vi "QPSK-PrError.vi"() -> ()   [LabVIEW 2019]
panel:
  out "Histogram":dynamicdata(graph)
  out "Sigma v.s. Eb/N0":cluster{"Y":dbl[], "Y":dbl[]}[](graph)=[{"Y"=[-4.0, -3.0, -2.0, -1.0, 0.0, 1.0, 2.0, 3.0, 4.0, 5.0, 6.0, 7.0, 8.0, 9.0, 10.0], "Y"=[0.22360679774997896, 0.22360679774997896, 0.22360679774997896, 0.22360679774997896, 0.22360679774997896, 0.22360679774997896, 0.22360679774997896, 0.22360679774997896, 0.22360679774997896, 0.22360679774997896, 0.22360679774997896, 0.22360679774997896, 0.22360679774997896, 0.22360679774997896, 0.22360679774997896]}, {"Y"=[-4.0, -3.0, -2.0, -1.0, 0.0, 1.0, 2.0, 3.0, 4.0, 5.0, 6.0, 7.0, 8.0, 9.0, 10.0], "Y"=[0.21946706488286016, 0.23428614669215203, 0.23032610126796704, 0.22554872351382088, 0.23060994158495868, 0.22799211096459765, 0.21892753075303117, 0.2211924581630937, 0.22337368763453955, 0.22373582900568173, 0.22421254226157725, 0.22347132110974322, 0.22376351654717402, 0.22364208288100582, 0.2235617892354569]}]
  out "Error v.s. Eb/N0":cluster{"Y":dbl[], "Y":dbl[]}[](graph)=[{"Y"=[-4.0, -3.0, -2.0, -1.0, 0.0, 1.0, 2.0, 3.0, 4.0, 5.0, 6.0, 7.0, 8.0, 9.0, 10.0], "Y"=[0.186113817483389, 0.15836831880959792, 0.13064448852282923, 0.10375909595340634, 0.0786496035251426, 0.05628195197654151, 0.03750612835892598, 0.022878407561085355, 0.012500818040737566, 0.005953867147778654, 0.0023882907809328045, 0.0007726748153784443, 0.00019090777407599314, 3.362722841961758e-05, 3.8721082155220345e-06]}, {"Y"=[-4.0, -3.0, -2.0, -1.0, 0.0, 1.0, 2.0, 3.0, 4.0, 5.0, 6.0, 7.0, 8.0, 9.0, 10.0], "Y"=[0.181126972072573, 0.18558256250571464, 0.1280283596632129, 0.09536252067637521, 0.07711725451253877, 0.05917048299972199, 0.03192674151170439, 0.018731266078510625, 0.014147931135755807, 0.006354844769778333, 0.0026571287865801377, 0.0008767372621810049, 0.00022169255900401932, 3.4706636641853096e-05, 4.417309341754243e-06]}]
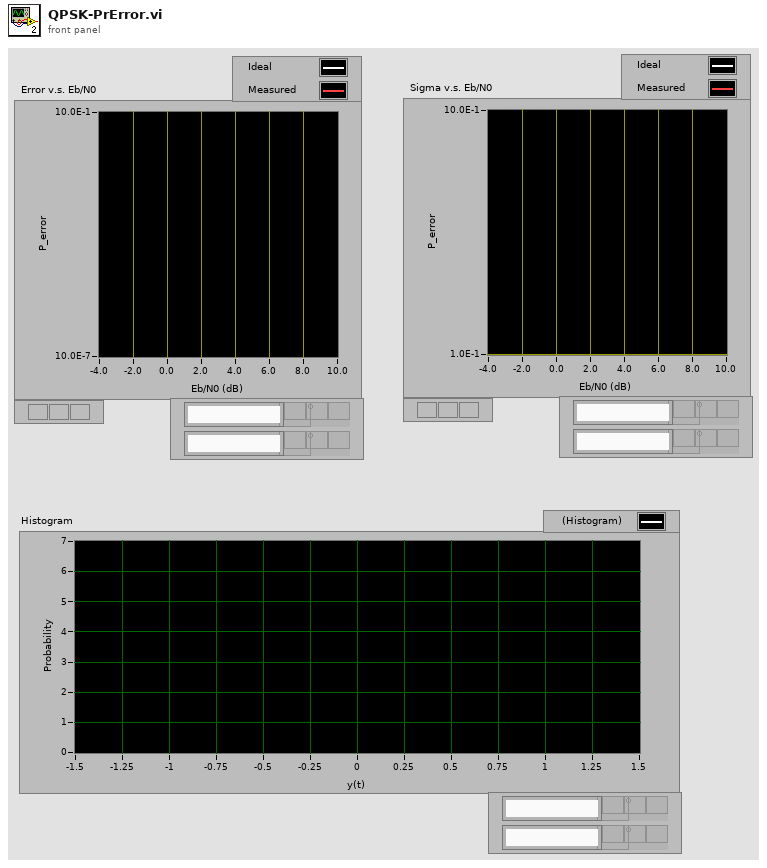
[diagram p1: front panel]
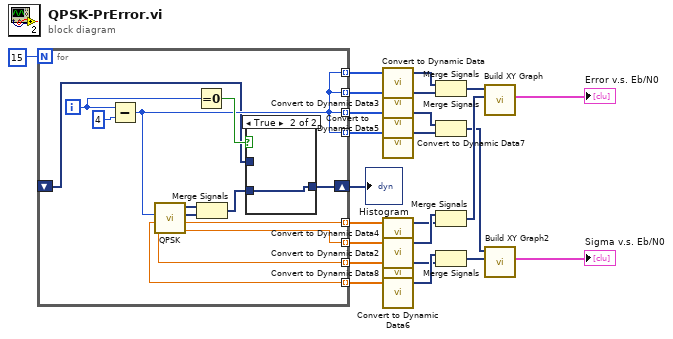
[diagram p0: block diagram]
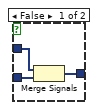
[diagram p2: hidden frame]
diagram:
  n1 = for {
    N: 15 -> [_]
    tunnel: [w32] -> w23 mode=indexing
    tunnel: [w31] -> w20 mode=indexing
    tunnel: [w32] -> w19 mode=indexing
    tunnel: [w30] -> w18 mode=indexing
    tunnel: [w33] -> w5 mode=indexing
    tunnel: [w34] -> w4 mode=indexing
    tunnel: [w32] -> w3 mode=indexing
    tunnel: [w32] -> w2 mode=indexing
    shift-right: [w25] -> w1
    shift-left: _ -> [w26]
    i -> [w36]
    n2 = Subtract(x=w36, y=4) -> (x-y=w32:i32)
    n3 = call "QPSK.vi"("ebn0"=w32) -> ("Pr(error) ideal"=w31:dbl, "Pr(error) measured"=w30:dbl, "Histogram (cos)"=w28:dynamicdata, "Histogram (sin)"=w29:dynamicdata, "Sigma_out (measured)"=w34:dbl, "Sigma_out (Ideal)"=w33:dbl)  [unwired: 3 in]
    n4 = Equal To 0?(x=w36) -> (x = 0?=w35:bool)
    n5 = Merge Signals(w29, w28) -> (w27:dynamicdata)
    n6 = case shown="True" w35 {
      tunnel: w27 -> [w40 w41]
      tunnel: w26 -> [w39 _]
      tunnel: [w38 w41] -> w25
      frame False {
        n7 = Merge Signals(w39, w40) -> (w38:dynamicdata)
      }
      frame True {
      }
    }
  }
  "Histogram" <- w1
  n8 = call "Convert to Dynamic Data"("Array"=w23) -> ("Dynamic Data Type"=w22:dynamicdata)  [unwired: 3 in]
  n9 = call "Convert to Dynamic Data3"("Array"=w19) -> ("Dynamic Data Type"=w16:dynamicdata)  [unwired: 3 in]
  n10 = call "Convert to Dynamic Data5"("Array"=w2) -> ("Dynamic Data Type"=w12:dynamicdata)  [unwired: 3 in]
  n11 = call "Convert to Dynamic Data7"("Array"=w3) -> ("Dynamic Data Type"=w9:dynamicdata)  [unwired: 3 in]
  n12 = call "Convert to Dynamic Data4"("Array"=w18) -> ("Dynamic Data Type"=w14:dynamicdata)  [unwired: 3 in]
  n13 = call "Convert to Dynamic Data2"("Array"=w20) -> ("Dynamic Data Type"=w21:dynamicdata)  [unwired: 3 in]
  n14 = call "Convert to Dynamic Data8"("Array"=w4) -> ("Dynamic Data Type"=w7:dynamicdata)  [unwired: 3 in]
  n15 = call "Convert to Dynamic Data6"("Array"=w5) -> ("Dynamic Data Type"=w11:dynamicdata)  [unwired: 3 in]
  n16 = Merge Signals(w22, w16) -> (w17:dynamicdata)
  n17 = Merge Signals(w12, w9) -> (w10:dynamicdata)
  n18 = Merge Signals(w21, w14) -> (w15:dynamicdata)
  n19 = Merge Signals(w11, w7) -> (w8:dynamicdata)
  n20 = call "Build XY Graph"("Y Input"=w15, "X Input"=w17) -> ("XY Graph"=→"Error v.s. Eb/N0":cluster{"X":dbl[], "Y":dbl[]}[])  [unwired: 8 in, 1 out]
  n21 = call "Build XY Graph2"("Y Input"=w8, "X Input"=w10) -> ("XY Graph"=→"Sigma v.s. Eb/N0":cluster{"X":dbl[], "Y":dbl[]}[])  [unwired: 8 in, 1 out]
